vi "PR_Francisco_Rocha.vi"() -> ()   [LabVIEW 2016]
uses:
  <vilib>/Utility/file.llb/Write Delimited Spreadsheet (DBL).vi
panel:
  in  "Ref. Mult":dbl
  in  "Ref. LockIn":dbl
  in  "referencia":dbl
  in  "lecturas":i32
  in  "file path (use dialog)":path
  in  "Incremento (nm)":sgl=600.001 format="%.3f"
  out "VISA resource name out 2":refnum<visa-resource-name>
  out "Longitud de \nonda actual":dbl
  in  "Longitud de onda\nfinal  (nm)":sgl=600.001 format="%.3f"
  out "PR":cluster{"array":dbl[], "array":dbl[]}(graph)
  out "R":cluster{"array":dbl[], "array":dbl[]}(graph)
  out "DeltaR":cluster{"array":dbl[], "array":dbl[]}(graph)
  in  "Longitud de onda\ninicial  (nm)":sgl=600.001 format="%.3f"
  in  "?":bool
  in  "error in (no error)":errorcluster
  out "error out":errorcluster
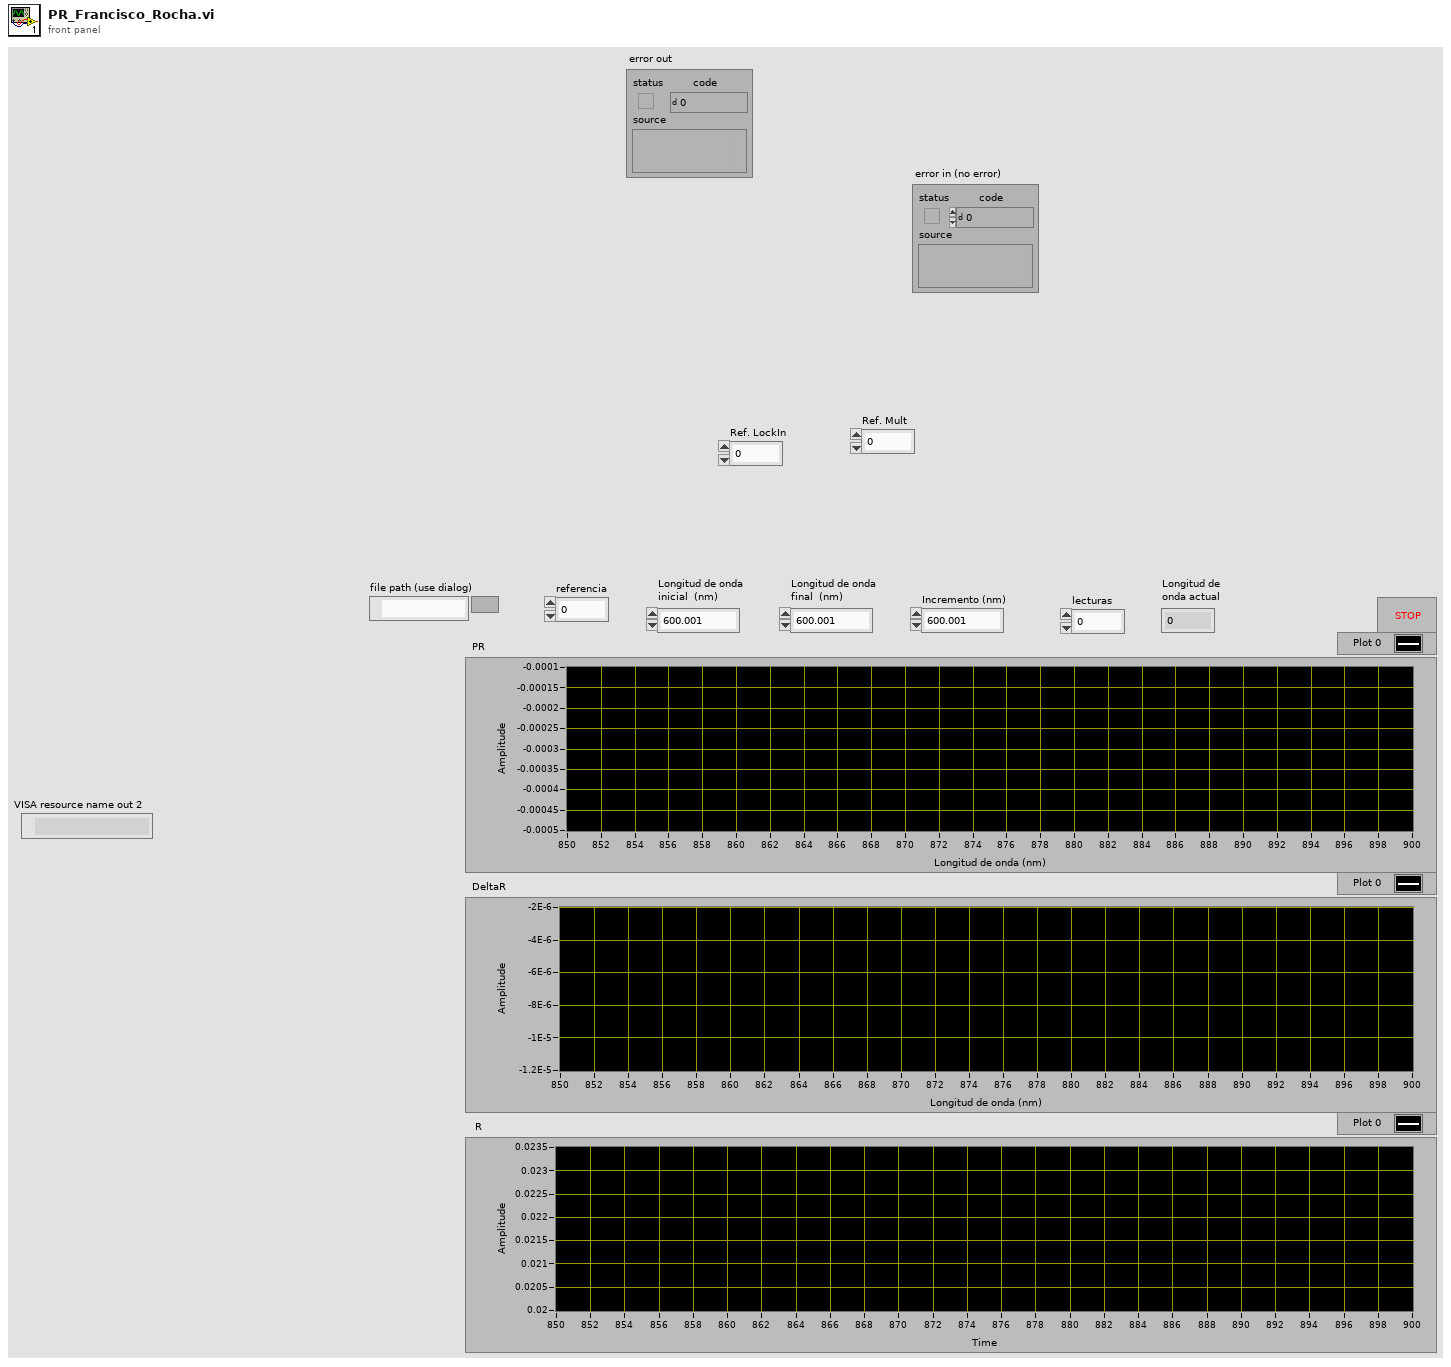
[diagram p1: front panel]
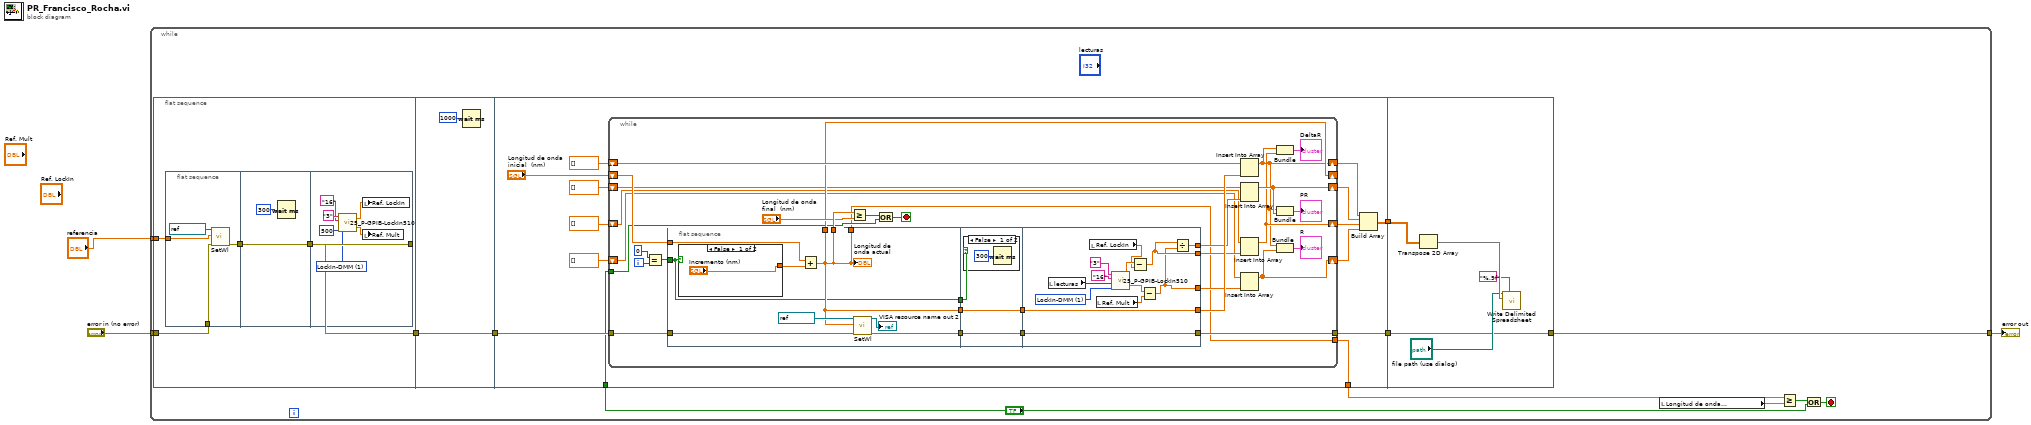
[diagram p0: block diagram]
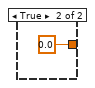
[diagram p2: hidden frame]
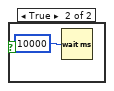
[diagram p3: hidden frame]
diagram:
  n1 = while {
    tunnel: "error in (no error)" -> [w7]
    tunnel: [w6] -> w2
    tunnel: "referencia" -> [w4]
    stop <- w10 stop-if-true
    n2 = flat-sequence {
      tunnel: w7 -> [w20]
      tunnel: [w19] -> w5
      tunnel: w4 -> [w16]
      tunnel: [w34] -> w8
      tunnel: w5 -> [w34]
      tunnel: w8 -> [w49]
      tunnel: "?" -> [w38]
      tunnel: [w48] -> w15
      tunnel: [w37] -> w14
      tunnel: [w36] -> w12
      tunnel: w15 -> [w112]
      tunnel: w14 -> [w115]
      tunnel: [w112] -> w6
      frame #0 {
        n3 = flat-sequence {
          tunnel: w20 -> [w23]
          tunnel: [w22] -> w18
          tunnel: w16 -> [w21]
          tunnel: w18 -> [w26]
          tunnel: [w26] -> w17
          tunnel: [w33] -> w19
          tunnel: w17 -> [w33]
          frame #0 {
            n4 = call "SetWl.vi"("VISA resource name"=refnum<visa-resource-name> "COM5", "Wavelength (nm)"=w21, "error in (no error)"=w23) -> ("error out"=w22:errorcluster)  [unwired: 15 in, 1 out]
          }
          frame #1 {
            n5 = Wait (ms)(milliseconds to wait=u32 300) -> ()  [unwired: 1 out]
          }
          frame #2 {
            w27 = u16 1 items=["LockIn", "LockIn-DMM"] ("Tipo")
            n6 = call "25_P-GPIB-LockIn510.vi"("Tipo"=w27, "Lecturas"=500, "P-DMM"="16", "P-LockIn"="3") -> ("DMM"=w30:dbl, "LockIn"=w29:dbl)
            n7 = local write "Ref. LockIn"(w29) -> ()
            n8 = local write "Ref. Mult"(w30) -> ()
          }
        }
      }
      frame #1 {
        n9 = Wait (ms)(milliseconds to wait=u32 1000) -> ()  [unwired: 1 out]
      }
      frame #2 {
        n10 = while {
          tunnel: w49 -> [w82]
          tunnel: [w81] -> w48
          shift-right: [w59] -> w42
          shift-left: dbl[] [] ("array") -> [w68]
          shift-right: [w67] -> _
          shift-left: "Longitud de onda\ninicial  (nm)" -> [w77]
          shift-right: [w61] -> w41
          shift-left: dbl[] [] ("array") -> [w65]
          shift-right: [w63] -> w40
          shift-left: dbl[] [] ("array") -> [w64]
          shift-right: [w58] -> w39
          shift-left: dbl[] [] ("array") -> [w66]
          tunnel: w38 -> [w56]
          tunnel: [w55] -> w36
          i -> [w80]
          stop <- w73 stop-if-true
          n11 = Equal?(x=0, y=w80) -> (x = y?=w78:bool)
          n12 = flat-sequence {
            tunnel: w82 -> [w90]
            tunnel: [w89] -> w54
            tunnel: w78 -> [w83]
            tunnel: w77 -> [w88]
            tunnel: [w84] -> w76
            tunnel: [w84] -> w52
            tunnel: [w84] -> w67
            tunnel: [w84] -> w55
            tunnel: [w83] -> w50
            tunnel: w54 -> [w95]
            tunnel: [w95] -> w53
            tunnel: w52 -> [w94]
            tunnel: [w94] -> w51
            tunnel: w50 -> [w93]
            tunnel: [w110] -> w81
            tunnel: w53 -> [w110]
            tunnel: [w106] -> w72
            tunnel: w51 -> [w106]
            tunnel: [w100] -> w71
            tunnel: [w103] -> w70
            tunnel: [w105] -> w69
            frame #0 {
              n13 = case shown="False" w83 {
                tunnel: ["Incremento (nm)" 0.0] -> w87
                frame False {
                }
                frame True {
                }
              }
              n14 = Add(x=w88, y=w87) -> (x+y=w84:dbl)
              "Longitud de \nonda actual" <- w84
              n15 = call "SetWl.vi"("VISA resource name"=refnum<visa-resource-name> "COM5", "Wavelength (nm)"=w84, "error in (no error)"=w90) -> ("VISA resource name out"=→"VISA resource name out 2":refnum<visa-resource-name>, "error out"=w89:errorcluster)  [unwired: 15 in]
            }
            frame #1 {
              n16 = case shown="False" w93 {
                frame False {
                  n17 = Wait (ms)(milliseconds to wait=u32 300) -> ()  [unwired: 1 out]
                }
                frame True {
                  n18 = Wait (ms)(milliseconds to wait=u32 10000) -> ()  [unwired: 1 out]
                }
              }
            }
            frame #2 {
              w104 = u16 1 items=["LockIn", "LockIn-DMM"] ("Tipo")
              n19 = local read "lecturas"() -> (w107:i32)
              n20 = local read "Ref. LockIn"() -> (w101:dbl)
              n21 = local read "Ref. Mult"() -> (w98:dbl)
              n22 = call "25_P-GPIB-LockIn510.vi"("Tipo"=w104, "Lecturas"=w107, "P-DMM"="16", "P-LockIn"="3") -> ("DMM"=w99:dbl, "LockIn"=w102:dbl)
              n23 = Subtract(x=w102, y=w101) -> (x-y=w103:dbl)
              n24 = Subtract(x=w99, y=w98) -> (x-y=w100:dbl)
              n25 = Divide(x=w103, y=w100) -> (x/y=w105:dbl)
            }
          }
          n26 = Greater Or Equal?(x=w76, y="Longitud de onda\nfinal  (nm)") -> (x >= y?=w74:bool)
          n27 = Or(x=w74, y=w56) -> (x .or. y?=w73:bool)
          n28 = Insert Into Array(array=w68, new element=w72) -> (w59:dbl[])  [unwired: 1 in]
          n29 = Insert Into Array(array=w64, new element=w69) -> (w63:dbl[])  [unwired: 1 in]
          n30 = Insert Into Array(array=w65, new element=w70) -> (w61:dbl[])  [unwired: 1 in]
          n31 = Insert Into Array(array=w66, new element=w71) -> (w58:dbl[])  [unwired: 1 in]
          n32 = Bundle("array"=w59, "array"=w61) -> (→"DeltaR":cluster{"array":dbl[], "array":dbl[]})  [unwired: 1 in]
          n33 = Bundle("array"=w59, "array"=w63) -> (→"PR":cluster{"array":dbl[], "array":dbl[]})  [unwired: 1 in]
          n34 = Bundle("array"=w59, "array"=w58) -> (→"R":cluster{"array":dbl[], "array":dbl[]})  [unwired: 1 in]
        }
        n35 = Build Array(w42, w40, w41, w39) -> (w37:dbl[][])
      }
      frame #3 {
        n36 = Transpose 2D Array(2D array=w115) -> (transposed array=w114:dbl[][])
        n37 = call-poly <vilib>:"Write Delimited Spreadsheet.vi"("file path (dialog if empty)"="file path (use dialog)", "format (%.3f)"="%.9f", "2D data"=w114) -> ()  [unwired: 11 in, 2 out]
      }
    }
    n38 = local read "Longitud de onda\nfinal  (nm)"() -> (w9:sgl)
    n39 = Greater Or Equal?(x=w12, y=w9) -> (x >= y?=w13:bool)
    n40 = Or(x=w13, y="?") -> (x .or. y?=w10:bool)
  }
  "error out" <- w2
